vi "Linear steps.vi"(1 "Steps":i32=201, 2 "To":dbl, 3 "From":dbl) -> (0 "Array":dbl[](array[numeric]))   [LabVIEW 2018]
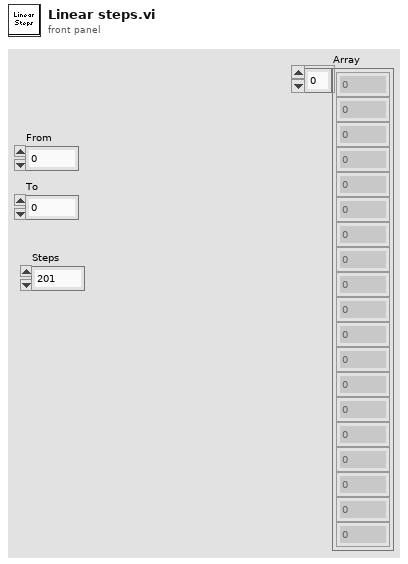
[diagram p1: front panel]
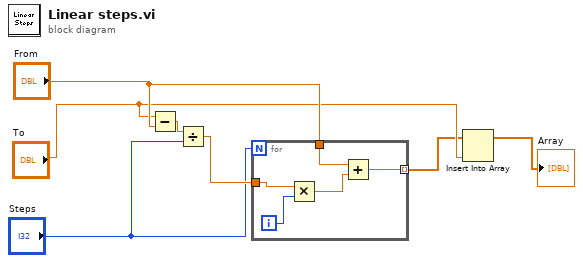
[diagram p0: block diagram]
diagram:
  n1 = Subtract(x="To", y="From") -> (x-y=w7:dbl)
  n2 = Divide(x=w7, y="Steps") -> (x/y=w6:dbl)
  n3 = for {
    N: "Steps" -> [_]
    tunnel: w6 -> [w12]
    tunnel: "From" -> [w9]
    tunnel: [w8] -> w2 mode=indexing
    i -> [w11]
    n4 = Multiply(x=w12, y=w11) -> (x*y=w10:dbl)
    n5 = Add(x=w9, y=w10) -> (x+y=w8:dbl)
  }
  n6 = Insert Into Array(array=w2, new element="To") -> (→"Array":dbl[])  [unwired: 1 in]
